vi "FPGA Main.vi"() -> ()   [LabVIEW 2019]
uses:
  Point Cluster.ctl
  <vilib>/rvi/Emulation/niFpgaGetClockAttributes.vi
  <vilib>/rvi/Emulation/niFpgaSctlEmulationGetInTimedLoop.vi
  <vilib>/rvi/Emulation/niFpgaEmulationReportErrorSimple.vi
  <vilib>/rvi/Emulation/niFpgaCriticalErrorInLSC.vi
  <vilib>/rvi/DataTransferAndStorage/Container/XNode/niFpgaContainer.xnode
  <vilib>/rvi/interface/RandomDataEmulation/nirviRandomDataFpgaReadWriteTemplate.vi
panel:
  out "IRQs":u32
  out "Cluster Result 2":T1[](array[typedef])
  in  "Cluster Sum 2":T1[](array[typedef])=[{"X"=0, "Y"=0}, {"X"=0, "Y"=0}]
  in  "Cluster Control 2":T1[](array[typedef])=[{"X"=0, "Y"=0}, {"X"=0, "Y"=0}]
  out "Cluster Result":T1
  in  "Cluster Sum":T1
  in  "Cluster Control":T1
  in  "Fxp Control":fxp<+/-,32,16>
  in  "Fxp Sum":fxp<+/-,32,16>
  out "Fxp Result":fxp<+/-,33,17> format="%.22g"
  in  "Fxp Control Array":fxp<+/-,32,16>[](array[numeric])=[0.0, 0.0, 0.0, 0.0]
  in  "Fxp Sum Array":fxp<+/-,32,16>[](array[numeric])=[0.0, 0.0, 0.0, 0.0]
  out "Fxp Result Array":fxp<+/-,33,17>[](array[numeric]) format="%.22g"
  in  "Sgl Control":sgl
  in  "Sgl Sum":sgl
  out "Sgl Result":sgl
  in  "Sgl Control Array":sgl[](array[numeric])=[0.0, 0.0, 0.0, 0.0]
  in  "Sgl Sum Array":sgl[](array[numeric])=[0.0, 0.0, 0.0, 0.0]
  out "Sgl Result Array":sgl[](array[numeric])
  in  "U8 Control Array":u8[](array[numeric])=[0, 0, 0, 0]
  in  "U8 Sum Array":u8[](array[numeric])=[0, 0, 0, 0]
  out "U8 Result Array":u8[](array[numeric])
  out "U8 Result":u8
  in  "U8 Sum":u8
  in  "U8 Control":u8
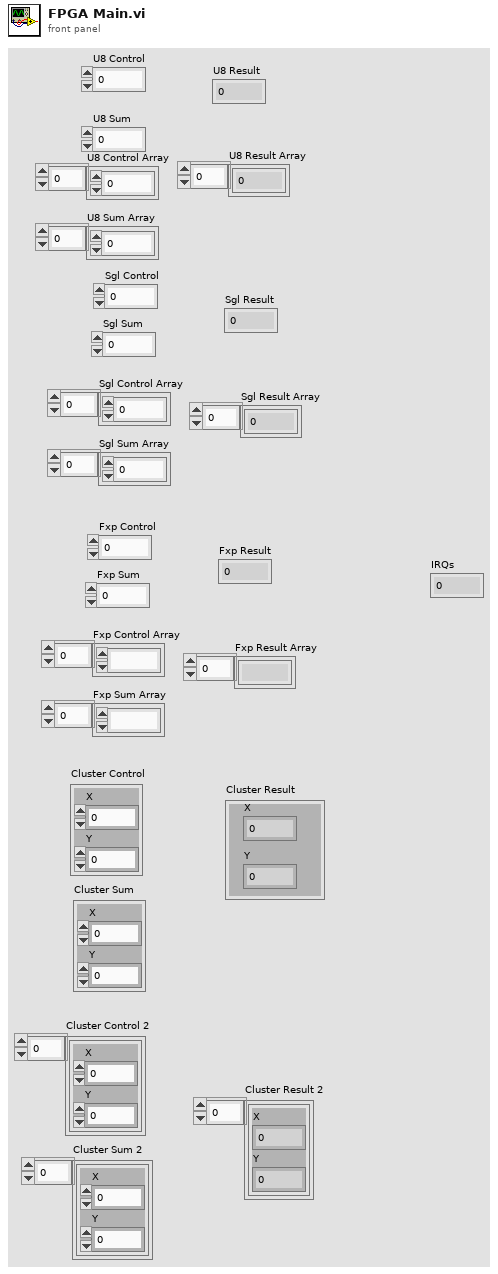
[diagram p1: front panel]
types:
  T1 = typedef "Point Cluster.ctl" = cluster{"X":i16, "Y":i16}
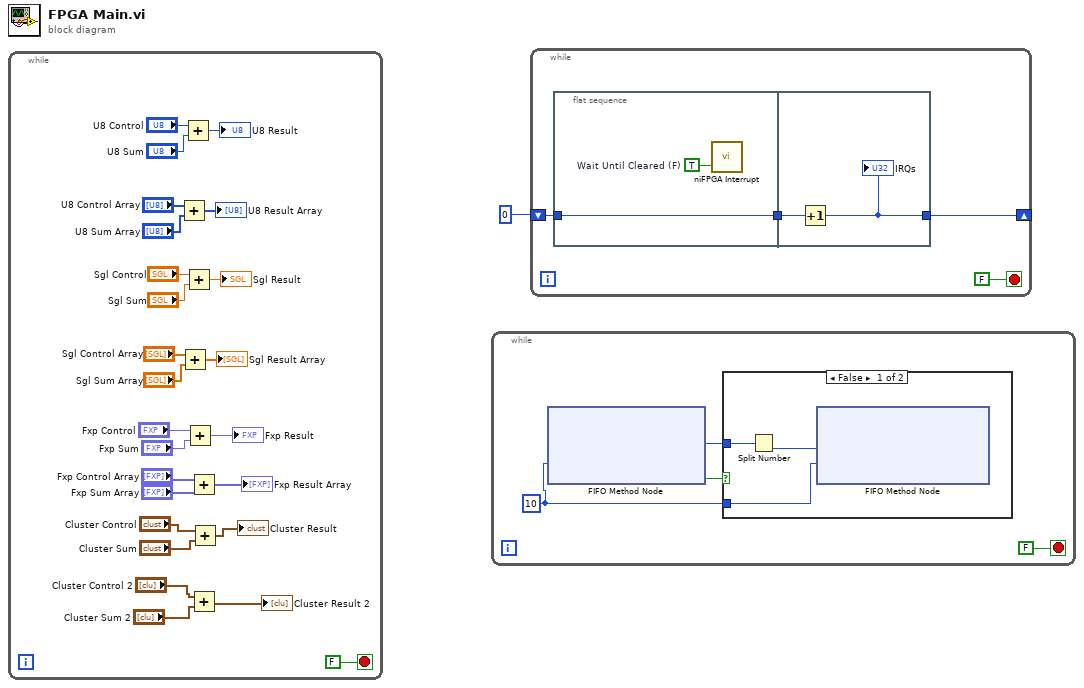
[diagram p0: block diagram]
diagram:
  n1 = while {
    stop <- FALSE stop-if-true
    n2 = Add(x="U8 Control Array", y="U8 Sum Array") -> (x+y=→"U8 Result Array":u8[])
    n3 = Add(x="Sgl Control Array", y="Sgl Sum Array") -> (x+y=→"Sgl Result Array":sgl[])
    n4 = Add(x="U8 Control", y="U8 Sum") -> (x+y=→"U8 Result":u8)
    n5 = Add(x="Sgl Control", y="Sgl Sum") -> (x+y=→"Sgl Result":sgl)
    n6 = Add(x="Fxp Control", y="Fxp Sum") -> (x+y=→"Fxp Result":fxp<+/-,33,17>)
    n7 = Add(x="Fxp Control Array", y="Fxp Sum Array") -> (x+y=→"Fxp Result Array":fxp<+/-,33,17>[])
    n8 = Add(x="Cluster Control 2", y="Cluster Sum 2") -> (x+y=→"Cluster Result 2":T1[])
    n9 = Add(x="Cluster Control", y="Cluster Sum") -> (x+y=→"Cluster Result":T1)
  }
  n10 = while {
    stop <- FALSE stop-if-true
    w28 = 10 ("Timeout")
    n11 = xnode ("FIFO Method Node")("Timeout"=w28) -> ("Element"=w30:u32, "Timed Out?"=w29:bool)  [unwired: 1 in, 1 out]
    n12 = case shown="False" w29 {
      tunnel: w30 -> [w33 _]
      tunnel: w28 -> [w31 _]
      frame False {
        n13 = Split Number(x=w33) -> (lo(x)=w32:u16)  [unwired: 1 out]
        n14 = xnode ("FIFO Method Node")("Element"=w32, "Timeout"=w31) -> ()  [unwired: 1 in, 2 out]
      }
      frame True {
      }
    }
  }
  n15 = while {
    shift-right: [w35] -> _
    shift-left: u32 0 -> [w36]
    stop <- FALSE stop-if-true
    n16 = flat-sequence {
      tunnel: [w38] -> w37
      tunnel: w36 -> [w38]
      tunnel: w37 -> [w41]
      tunnel: [w40] -> w35
      frame #0 {
        w39 = TRUE  # Wait Until Cleared (F)
        n17 = call <vilib>:"niFPGA Interrupt.vi"("Wait Until Cleared (F)"=w39) -> ()  [unwired: 2 in]
      }
      frame #1 {
        n18 = Increment(x=w41) -> (x+1=w40:u32)
        "IRQs" <- w40
      }
    }
  }
